vi "Unwrap1.vi"(1 "Numeric 2":dbl) -> (0 "Numeric":dbl)   [LabVIEW 2010]
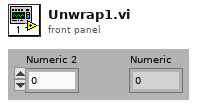
[diagram p1: front panel]
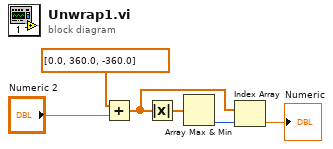
[diagram p0: block diagram]
diagram:
  n1 = Add(x=dbl[] [0.0, 360.0, -360.0], y="Numeric 2") -> (x+y=w3:dbl[])
  n2 = Absolute Value(x=w3) -> (abs(x)=w2:dbl[])
  n3 = Array Max & Min(array=w2) -> (min index (indices)=w4:i32)  [unwired: 3 out]
  n4 = Index Array(array=w3, index=w4) -> (element=→"Numeric":dbl)
